vi "ParseArray.vi"(8 "error in (no error)":errorcluster, 10 "Index In":i32, 11 "JSON String":string) -> (0 "error out":errorcluster, 2 "Index Out":i32, 3 "JSON Tree":variant)   [LabVIEW 2015, in "i3-json.lvlib"]
doc: "Use this template to build a VI to use as a subVI."
uses:
  i3-json.lvlib
  JSON Types/JSON Type.ctl
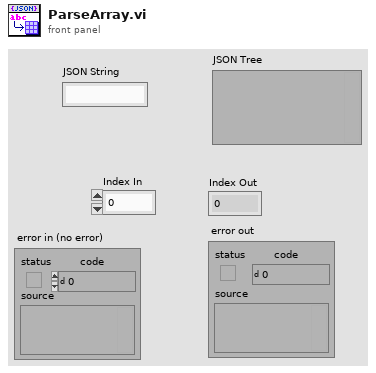
[diagram p1: front panel]
types:
  T1 = typedef "i3-json.lvlib/JSON Type.ctl" = enum8{"JSON Compatible", "JSON Array", "JSON Object", "JSON Null", "Double", "String", "Boolean", "Unknown"}
  T2 = typedef "i3-json.lvlib/Token.ctl" = enum16{"NONE", "CURLY_OPEN", "CURLY_CLOSE", "SQUARED_OPEN", "SQUARED_CLOSE", "COLON", "COMMA", "STRING", "NUMBER", "TRUE", "FALSE", "NULL"}
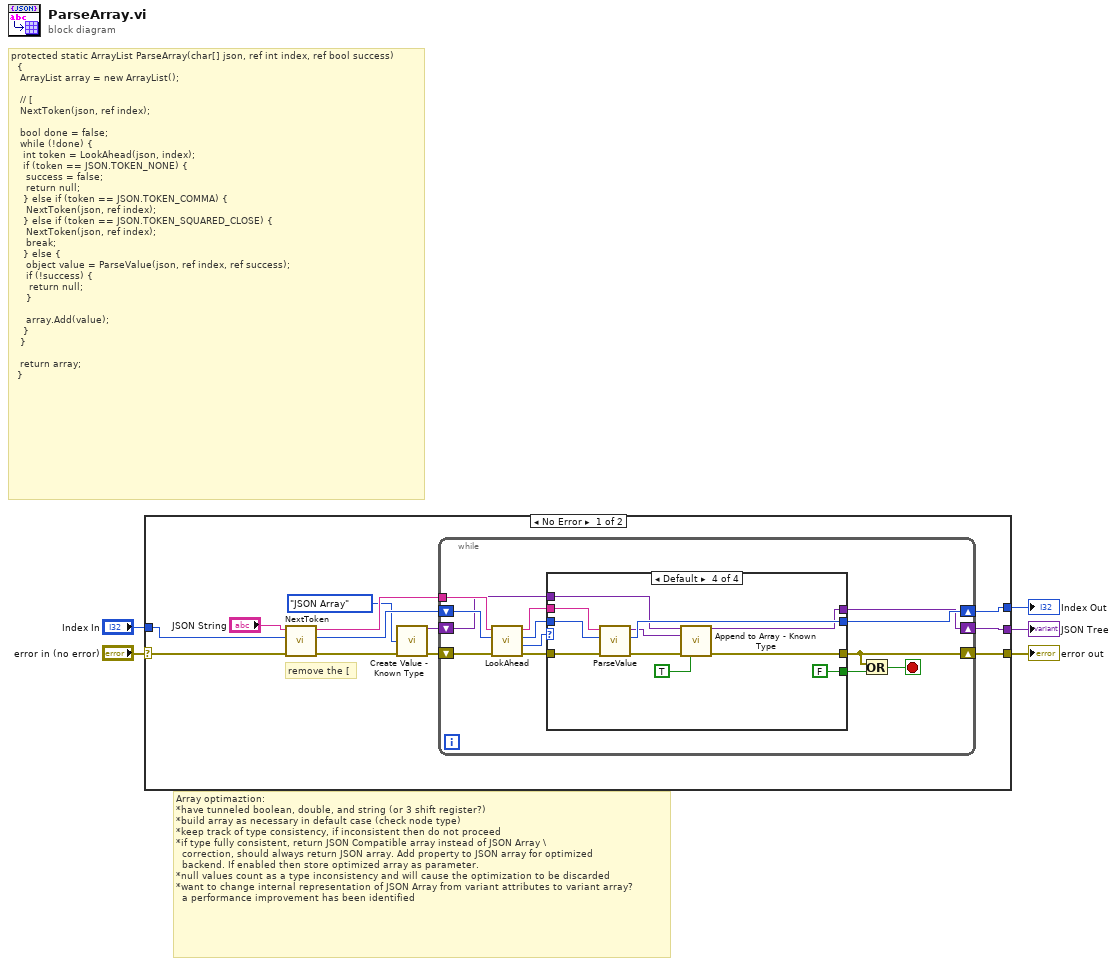
[diagram p0: block diagram]
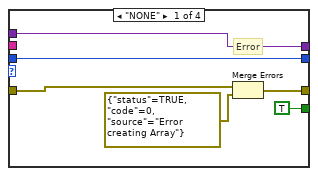
[diagram p2: hidden frame]
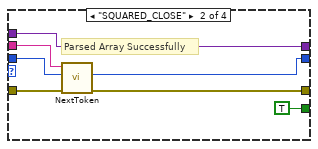
[diagram p3: hidden frame]
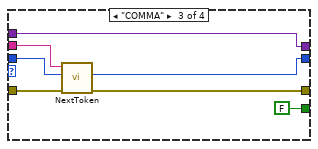
[diagram p4: hidden frame]
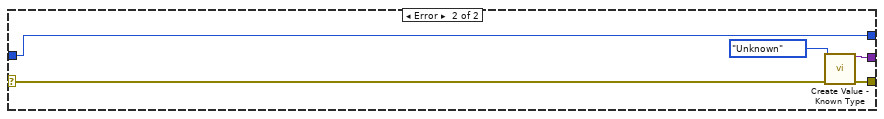
[diagram p5: hidden frame]
diagram:
  # "Array optimaztion:\n*have tunneled boolean, double, and string (or 3 shift register?)\n*build array as necessary in default case (check node type)\n*keep track of type consistency, if inconsistent then do not proceed\n*if type fully consistent, return JSON Compatible array instead of JSON Array \\\n  correction, should always return JSON array. Add property to JSON array for optimized\n  backend. If enabled then store optimized array as parameter.\n*null values count as a type inconsistency and will cause the optimization to be discarded\n*want to change internal representation of JSON Array from variant attributes to variant array?\n  a performance improvement has been identified"
  # "protected static ArrayList ParseArray(char[] json, ref int index, ref bool success)\n\t\t{\n\t\t\tArrayList array = new ArrayList();\n\n\t\t\t// [\n\t\t\tNextToken(json, ref index);\n\n\t\t\tbool done = false;\n\t\t\twhile (!done) {\n\t\t\t\tint token = LookAhead(json, index);\n\t\t\t\tif (token == JSON.TOKEN_NONE) {\n\t\t\t\t\tsuccess = false;\n\t\t\t\t\treturn null;\n\t\t\t\t} else if (token == JSON.TOKEN_COMMA) {\n\t\t\t\t\tNextToken(json, ref index);\n\t\t\t\t} else if (token == JSON.TOKEN_SQUARED_CLOSE) {\n\t\t\t\t\tNextToken(json, ref index);\n\t\t\t\t\tbreak;\n\t\t\t\t} else {\n\t\t\t\t\tobject value = ParseValue(json, ref index, ref success);\n\t\t\t\t\tif (!success) {\n\t\t\t\t\t\treturn null;\n\t\t\t\t\t}\n\n\t\t\t\t\tarray.Add(value);\n\t\t\t\t}\n\t\t\t}\n\n\t\t\treturn array;\n\t\t}"
  n1 = case shown="No Error" "error in (no error)" {
    selector: "error in (no error)" -> [w17 w66]
    tunnel: [w6 w65] -> w4
    tunnel: "Index In" -> [w16 w64]
    tunnel: [w8 w64] -> w2
    tunnel: [w7 w63] -> w1
    frame No Error {
      # "remove the ["
      n2 = call "NextToken.vi"("error in (no error)"=w17, "Index In"=w16, "JSON String"="JSON String") -> ("error out"=w12:errorcluster, "Index Out"=w14:i32, "JSON String Passthrough"=w13:string)  [unwired: 4 in, 1 out]
      n3 = call "Create Value - Known Type.vi"("JSON Type"=JSON_Type."JSON Array", "error in (no error)"=w12) -> ("JSON Tree"=w10:variant, "error out"=w11:errorcluster)  [unwired: 12 in]
      n4 = while {
        shift-right: [w23] -> w8
        shift-left: w14 -> [w29]
        tunnel: w13 -> [w28]
        shift-right: [w22] -> w7
        shift-left: w10 -> [w21]
        shift-right: [w18] -> w6
        shift-left: w11 -> [w30]
        stop <- w19 stop-if-true
        n5 = call "LookAhead.vi"("error in (no error)"=w30, "Index"=w29, "JSON String"=w28) -> ("error out"=w26:errorcluster, "TOKEN"=w27:T2, "Index Passthrough"=w25:i32, "JSON String Passthrough"=w24:string)  [unwired: 4 in]
        n6 = case shown="Default" w27 {
          tunnel: w26 -> [w32 w43 w48 w61]
          tunnel: [TRUE TRUE FALSE FALSE] -> w20
          tunnel: w25 -> [w35 w42 w49 w60]
          tunnel: w24 -> [_ w41 w50 w59]
          tunnel: [w35 w39 w46 w58] -> w23
          tunnel: [w34 w38 w45 w52] -> w22
          tunnel: w21 -> [w34 w38 w45 w53]
          tunnel: [w33 w40 w47 w51] -> w18
          frame "NONE" {
            # "Error"
            n7 = Merge Errors(w32, errorcluster {"status"=TRUE, "code"=0, "source"="Error creating Array"} ("error out")) -> (w33:errorcluster)
          }
          frame "SQUARED_CLOSE" {
            # "Parsed Array Successfully"
            n8 = call "NextToken.vi"("error in (no error)"=w43, "Index In"=w42, "JSON String"=w41) -> ("error out"=w40:errorcluster, "Index Out"=w39:i32)  [unwired: 4 in, 2 out]
          }
          frame "COMMA" {
            n9 = call "NextToken.vi"("error in (no error)"=w48, "Index In"=w49, "JSON String"=w50) -> ("error out"=w47:errorcluster, "Index Out"=w46:i32)  [unwired: 4 in, 2 out]
          }
          frame Default {
            n10 = call "ParseValue.vi"("error in (no error)"=w61, "Index In"=w60, "JSON String"=w59) -> ("error out"=w56:errorcluster, "Index Out"=w58:i32, "JSON Tree"=w55:variant)  [unwired: 6 in]
            n11 = call "Append to Array - Known Type.vi"("JSON Tree in (JSON Array)"=w53, "Value"=w55, "error in (no error)"=w56, "Add Parameter as JSON Tree?"=TRUE) -> ("JSON Tree out (JSON Array)"=w52:variant, "error out"=w51:errorcluster)  [unwired: 10 in]
          }
        }
        n12 = Or(x=w18, y=w20) -> (x .or. y?=w19:bool)
      }
    }
    frame Error {
      n13 = call "Create Value - Known Type.vi"("JSON Type"=JSON_Type."Unknown", "error in (no error)"=w66) -> ("JSON Tree"=w63:variant, "error out"=w65:errorcluster)  [unwired: 12 in]
    }
  }
  "error out" <- w4
  "Index Out" <- w2
  "JSON Tree" <- w1
